vi "Rocket Dynamics (SubVI).vi"(0 "TVA":T5, 2 "Data":dbl[][](array[numeric]), 3 "V_Wind [m/s]":dbl[][](array[numeric]), 4 "Vehicle Param":T4, 5 "Time":T3, 6 "Rotation":T2, 7 "Position":T1, 11 "Fe_data":dbl[](array[numeric])) -> (23 "output Rocket Dynamics":T6)   [LabVIEW 2017]
panel:
  out "q_aux":dbl[](array[numeric])
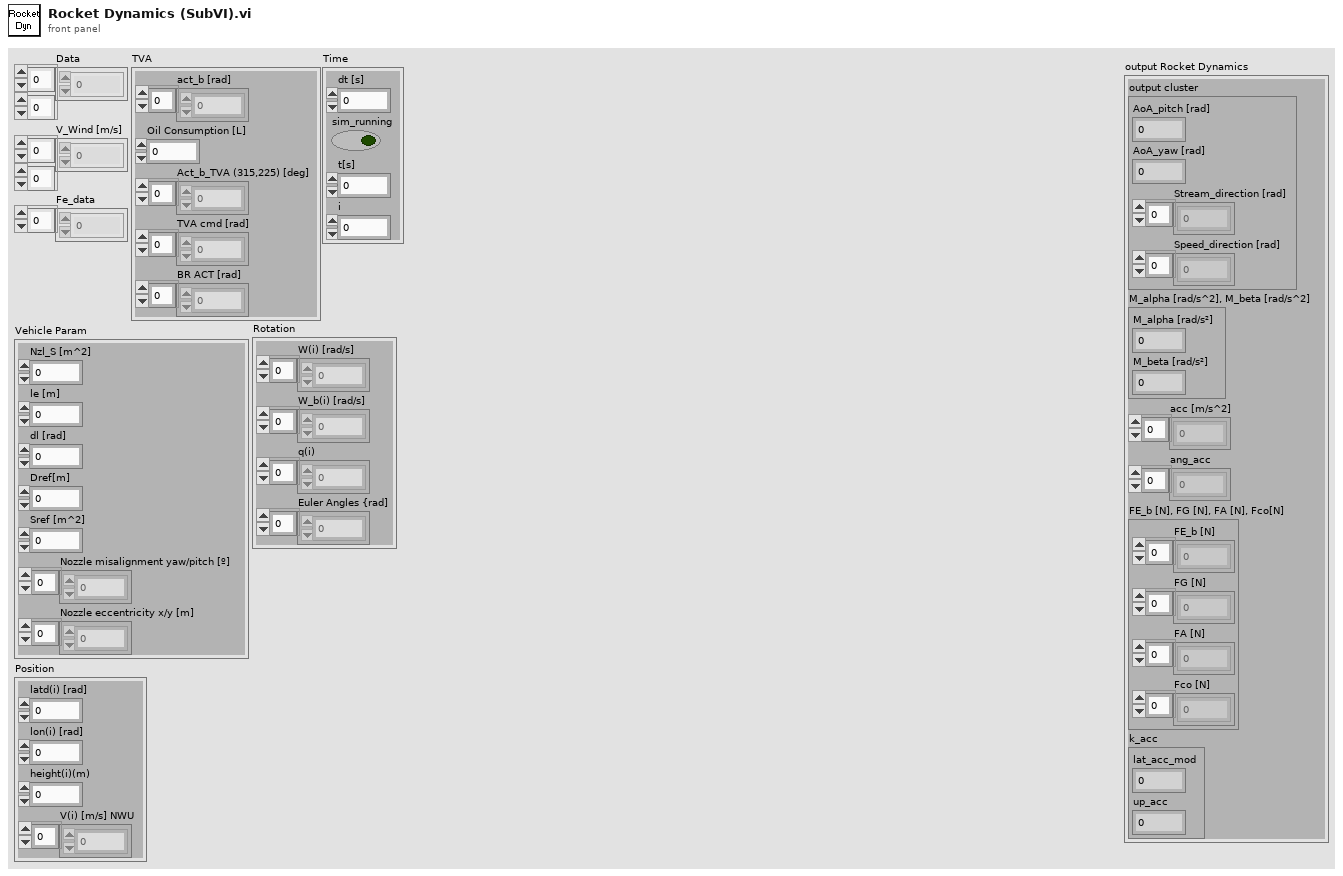
[diagram p1: front panel]
types:
  T1 = cluster{"latd(i) [rad]":dbl, "lon(i) [rad]":dbl, "height(i)(m)":dbl, "V(i) [m/s] NWU":dbl[]}
  T2 = cluster{"W(i) [rad/s]":dbl[], "W_b(i) [rad/s]":dbl[], "q(i)":dbl[], "Euler Angles {rad]":dbl[]}
  T3 = cluster{"dt [s]":dbl, "sim_running":bool, "t[s]":dbl, "i":i32}
  T4 = cluster{"Nzl_S [m^2]":dbl, "le [m]":dbl, "dl [rad]":dbl, "Dref[m]":dbl, "Sref [m^2]":dbl, "Nozzle misalignment yaw/pitch [º]":dbl[], "Nozzle eccentricity x/y [m]":dbl[]}
  T5 = cluster{"act_b [rad]":dbl[], "Oil Consumption [L]":dbl, "Act_b_TVA (315,225) [deg]":dbl[], "TVA cmd [rad]":dbl[], "BR ACT [rad]":dbl[]}
  T6 = cluster{"output cluster":cluster{"AoA_pitch [rad]":dbl, "AoA_yaw [rad]":dbl, "Stream_direction [rad]":dbl[], "Speed_direction [rad]":dbl[]}, "M_alpha [rad/s^2], M_beta [rad/s^2]":cluster{"M_alpha [rad/s²]":dbl, "M_beta [rad/s²]":dbl}, "acc [m/s^2]":dbl[], "ang_acc":dbl[], "FE_b [N], FG [N], FA [N], Fco[N]":cluster{"FE_b [N]":dbl[], "FG [N]":dbl[], "FA [N]":dbl[], "Fco [N]":dbl[]}, "k_acc":cluster{"lat_acc_mod":dbl, "up_acc":dbl}}
  T7 = cluster{"AoA_pitch [rad]":dbl, "AoA_yaw [rad]":dbl, "Stream_direction [rad]":dbl[], "Speed_direction [rad]":dbl[]}
  T8 = cluster{"Pdin [Pa]":dbl, "Patm [Pa]":dbl, "Temp [K]":dbl, "air flow velocity [m/s]":dbl}
  T9 = cluster{"AoA_pitch [rad]":dbl, "AoA_yaw [rad]":dbl, "Stream_direction [rad]":dbl[]}
  T10 = cluster{"M_alpha [rad/s²]":dbl, "M_beta [rad/s²]":dbl}
  T11 = cluster{"FE_b [N]":dbl[], "FG [N]":dbl[], "FA [N]":dbl[], "Fco [N]":dbl[]}
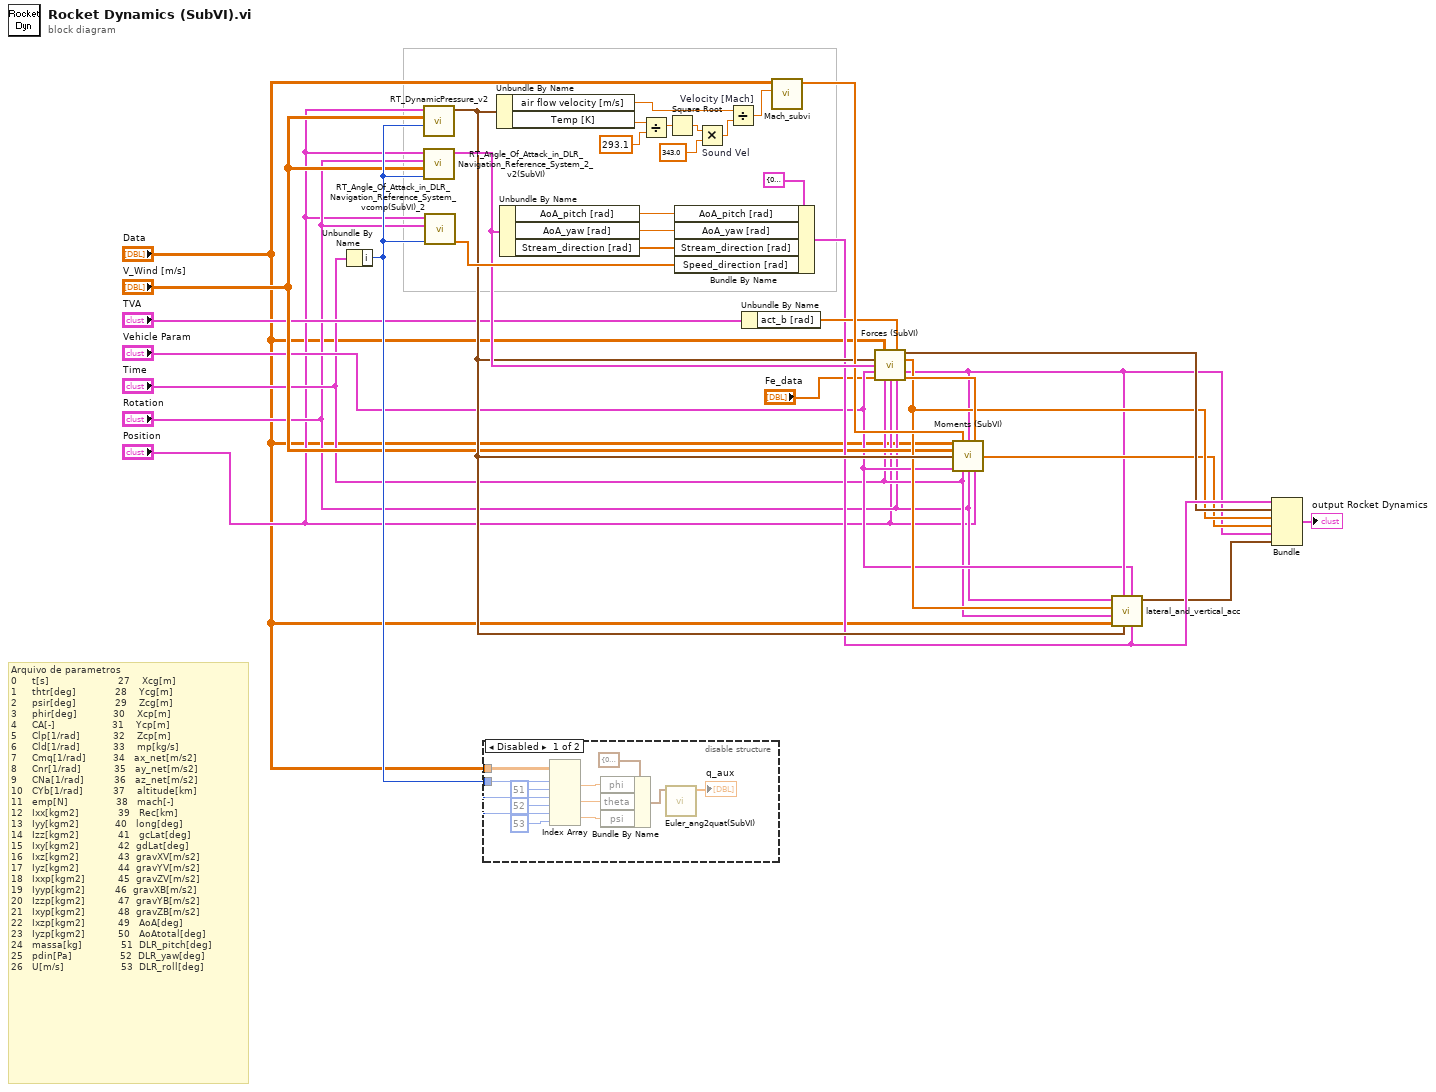
[diagram p0: block diagram]
diagram:
  # "Arquivo de parametros\n0     t[s]                       27    Xcg[m] \n1     thtr[deg]             28    Ycg[m]\n2     psir[deg]             29    Zcg[m]  \n3     phir[deg]            30    Xcp[m]       \n4     CA[-]                   31    Ycp[m]        \n5     Clp[1/rad]           32    Zcp[m]     \n6     Cld[1/rad]           33    mp[kg/s]        \n7     Cmq[1/rad]         34   ax_net[m/s2]         \n8     Cnr[1/rad]           35   ay_net[m/s2]      \n9     CNa[1/rad]          36   az_net[m/s2]      \n10   CYb[1/rad]          37    altitude[km]       \n11   emp[N]                38   mach[-]     \n12   Ixx[kgm2]             39   Rec[km]     \n13   Iyy[kgm2]            40   long[deg]     \n14   Izz[kgm2]             41   gcLat[deg]        \n15   Ixy[kgm2]             42  gdLat[deg]       \n16   Ixz[kgm2]             43  gravXV[m/s2]  \n17   Iyz[kgm2]             44  gravYV[m/s2]     \n18   Ixxp[kgm2]           45  gravZV[m/s2]         \n19   Iyyp[kgm2]          46  gravXB[m/s2]         \n20   Izzp[kgm2]           47  gravYB[m/s2]         \n21   Ixyp[kgm2]           48  gravZB[m/s2]           \n22   Ixzp[kgm2]           49   AoA[deg]             \n23   Iyzp[kgm2]           50   AoAtotal[deg]       \n24   massa[kg]             51  DLR_pitch[deg]    \n25   pdin[Pa]                52  DLR_yaw[deg]  \n26   U[m/s]                   53  DLR_roll[deg]"
  n1 = Unbundle By Name("Time") -> ("i"=w17:i32)
  n2 = call "RT_DynamicPressure_v2.vi"("i"=w17, "V_wind [m/s]"="V_Wind [m/s]", "output cluster 2"="Position") -> ("output cluster"=w16:T8)  [unwired: 8 in]
  n3 = call "RT_Angle_Of_Attack_in_DLR_Navigation_Reference_System_2_v2(SubVI).vi"("i"=w17, "V_wind [m/s]"="V_Wind [m/s]", "Rotation"="Rotation", "output cluster 2"="Position") -> ("output cluster"=w29:T9)  [unwired: 7 in]
  n4 = call "RT_Angle_Of_Attack_in_DLR_Navigation_Reference_System_vcomp(SubVI)_2.vi"("i"=w17, "Rotation"="Rotation", "input cluster"="Position") -> ("Speed_direction [rad]"=w34:dbl[])  [unwired: 6 in, 2 out]
  n5 = disable-structure shown="Disabled" {
    disable-tunnel: "Data" -> [w45 _]
    disable-tunnel: w17 -> [w44 _]
    frame Disabled {
      n6 = Index Array(array=w45, index (row) #1=w44, index (col) #1=51 ("disabled index (col)"), index (row) #2=w44, index (col) #2=52 ("disabled index (col)"), index (row) #3=w44, index (col) #3=53 ("disabled index (col)")) -> (element #1=w39:dbl, element #2=w38:dbl, element #3=w37:dbl)
      n7 = Bundle By Name(cluster=cluster{"phi":dbl, "theta":dbl, "psi":dbl} {"phi"=0.0, "theta"=0.0, "psi"=0.0} ("Euler Angles [deg]"), "phi"=w39, "theta"=w38, "psi"=w37) -> (w36:cluster{"phi":dbl, "theta":dbl, "psi":dbl})
      n8 = call "Euler_ang2quat(SubVI).vi"("Euler Angles [deg]"=w36) -> ("Quaternions"=→"q_aux":dbl[])  [unwired: 10 in]
    }
    frame Enabled {
    }
  }
  n9 = Unbundle By Name(w16) -> ("air flow velocity [m/s]"=w25:dbl, "Temp [K]"=w28:dbl)
  n10 = Unbundle By Name(w29) -> ("AoA_pitch [rad]"=w30:dbl, "AoA_yaw [rad]"=w31:dbl, "Stream_direction [rad]"=w32:dbl[])
  n11 = Divide(x=w28, y=293.1) -> (x/y=w20:dbl)
  n12 = Square Root(x=w20) -> (sqrt(x)=w21:dbl)
  n13 = Bundle By Name(cluster=T7 {"AoA_pitch [rad]"=0.0, "AoA_yaw [rad]"=0.0, "Stream_direction [rad]"=[], "Speed_direction [rad]"=[]} ("output cluster"), "AoA_pitch [rad]"=w30, "AoA_yaw [rad]"=w31, "Stream_direction [rad]"=w32, "Speed_direction [rad]"=w34) -> (w15:T7)
  n14 = Multiply "Sound Vel"(x=w21, y=343.0 ("x")) -> (x*y=w23:dbl)
  n15 = Divide "Velocity [Mach]"(x=w25, y=w23) -> (x/y=w24:dbl)
  n16 = Unbundle By Name("TVA") -> ("act_b [rad]"=w18:dbl[])
  n17 = call "Mach_subvi.vi"("Mach_IN"=w24, "Mach_File"="Data") -> ("OUT_Interp"=w27:dbl[])  [unwired: 9 in]
  n18 = call "Forces (SubVI).vi"("Data"="Data", "act_b"=w18, "Pdin [Pa], Patm [Pa], Temp [K], airflow velocity [m/s]"=w16, "AoA_pitch [rad], AoA_yaw [rad], Stream direction [rad]"=w29, "Vehicle Parameters"="Vehicle Param", "Fe_data"="Fe_data", "i, sim_running, t[s], dt[s]"="Time", "V(i) [m/s] NWU, latd(i) [rad], lon(i) [rad], height(i) [m]"="Position", "Rotation"="Rotation") -> ("M_alpha [rad/s^2], M_beta [rad/s^2]"=w14:T10, "acc [m/s^2]"=w13:dbl[], "FE_b [N], FG [N], FA [N], Fco[N]"=w11:T11, "FE [N]"=w26:dbl[])  [unwired: 3 in]
  n19 = call "Moments (SubVI).vi"("Data"="Data", "OUT_Interp"=w27, "FE_b [N], FG [N], FA [N], Fco[N]"=w11, "FE [N]"=w26, "V_Wind [m/s]"="V_Wind [m/s]", "Pdin [Pa], Patm [Pa], Temp [K], airflow velocity [m/s]"=w16, "Vehicle Parameters"="Vehicle Param", "i, sim_running, t[s], dt[s]"="Time", "Rotation"="Rotation", "V(i) [m/s] NWU, latd(i) [rad], lon(i) [rad], height(i) [m]"="Position") -> ("ang_acc"=w12:dbl[])  [unwired: 5 in]
  n20 = call "lateral_and_vertical_acc.vi"("Aerodyn output"=w15, "Vehicle Param"="Vehicle Param", "Pdyn2"=w16, "FE_b [N], FG [N], FA [N], Fco[N]"=w11, "Data"="Data", "Time"="Time", "acc [m/s^2]"=w13, "Rotation"="Rotation") -> ("k_acc"=w10:cluster{"lat_acc_mod":dbl, "up_acc":dbl})  [unwired: 3 in]
  n21 = Bundle("output cluster"=w15, "M_alpha [rad/s^2], M_beta [rad/s^2]"=w14, "acc [m/s^2]"=w13, "ang_acc"=w12, "FE_b [N], FG [N], FA [N], Fco[N]"=w11, "k_acc"=w10) -> (→"output Rocket Dynamics":T6)  [unwired: 1 in]
